vi "Read DriveCommand.vi"(8 "error in (no error)":errorcluster, 11 "DriveData in":refnum<class "DriveData.lvclass">) -> (0 "error out":errorcluster, 2 "DriveCommand":T1, 3 "DriveData out":refnum<class "DriveData.lvclass">)   [LabVIEW 2017]
uses:
  DriveData.lvclass
  R:/Documents/github/FRC4080/2018-robot-main/SubsystemData/SubsystemData.lvclass
  DriveCommand.ctl
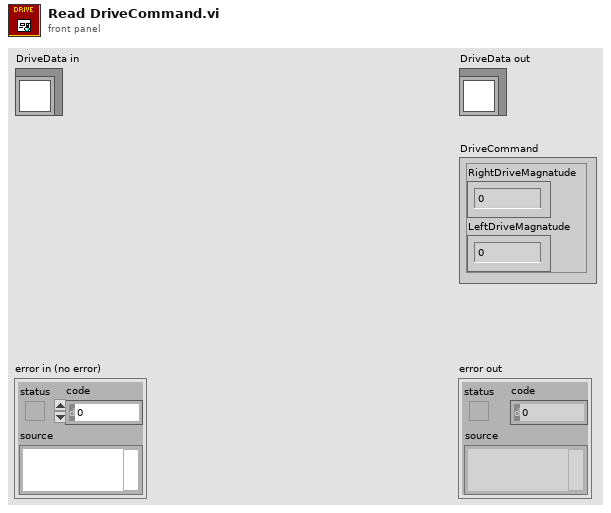
[diagram p1: front panel]
types:
  T1 = typedef "DriveData.lvclass/DriveCommand.ctl" = cluster{"RightDriveMagnatude":dbl, "LeftDriveMagnatude":dbl}
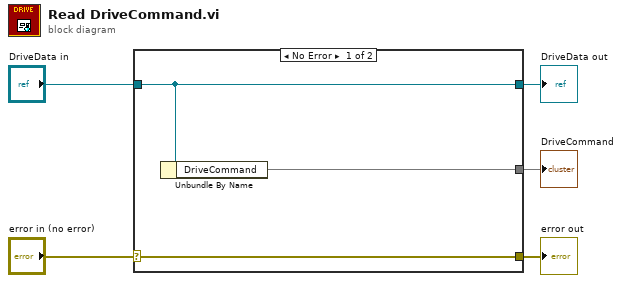
[diagram p0: block diagram]
diagram:
  n1 = case shown="No Error" "error in (no error)" {
    selector: "error in (no error)" -> [w8 w9]
    tunnel: [w8 w9] -> w4
    tunnel: [w7 w10] -> w2
    tunnel: "DriveData in" -> [w7 w10]
    tunnel: [w6 _] -> w1
    frame No Error {
      n2 = Unbundle By Name(w7) -> ("DriveCommand"=w6)
    }
    frame Error {
    }
  }
  "error out" <- w4
  "DriveData out" <- w2
  "DriveCommand" <- w1
